vi "to_number.vi"(8 "error in (no error)":errorcluster, 11 "MeasurementResult in":refnum<class "MeasurementResult.lvclass">) -> (0 "error out":errorcluster, 2 "outputs":dbl[](array[numeric]), 3 "MeasurementResult out":refnum<class "MeasurementResult.lvclass">)   [LabVIEW 2017, in "MeasurementResult.lvclass"]
doc: "Convert he measurement result to numbers"
uses:
  MeasurementResult.lvclass
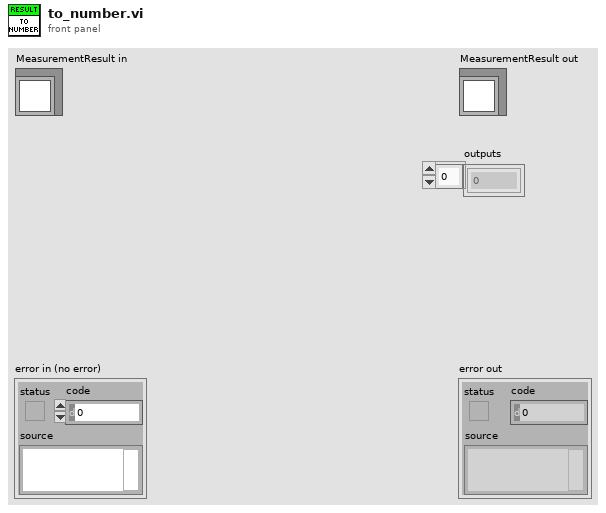
[diagram p1: front panel]
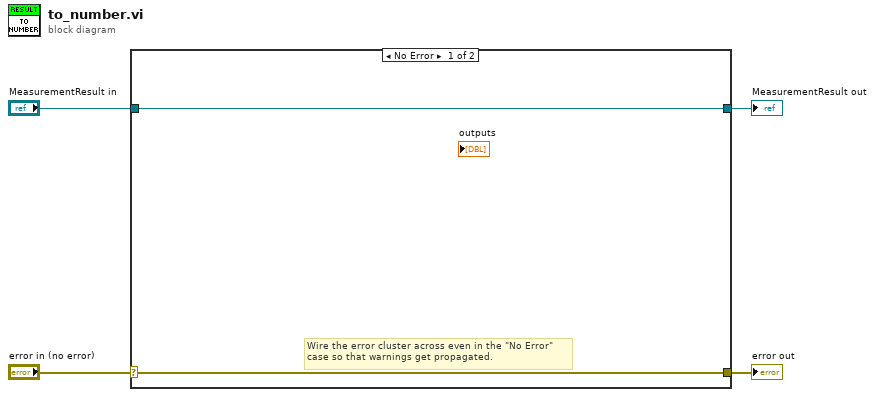
[diagram p0: block diagram]
diagram:
  n1 = case shown="No Error" "error in (no error)" {
    selector: "error in (no error)" -> [w5 w8]
    tunnel: [w5 w8] -> w3
    tunnel: [w6 w7] -> w1
    tunnel: "MeasurementResult in" -> [w6 w7]
    frame No Error {
      # "Wire the error cluster across even in the \"No Error\"\ncase so that warnings get propagated."
    }
    frame Error {
    }
  }
  "error out" <- w3
  "MeasurementResult out" <- w1
